vi "Clear Mutation History.vi"   [LabVIEW 2019]
uses:
  <vilib>/Utility/EditLVLibs/Edit LVLibs.lvlib
types:
  T1 = typedef "Edit LVLibs.lvlib/Mutation History.ctl" = T2[]
  T2 = typedef "Edit LVLibs.lvlib/Mutation Record.ctl" = cluster{"Library Version":T3, "Old Name Index":u8, "Class Default Data":variant, "Cluster Order Map":u32[], "Parent Name":string, "Parent Path":path, "LabVIEW Version":u32, "User Comments":string, "Mutation Flags":u8, "Parent Old Name Index":u8, "Parent Levels Added":u16, "Parent Levels Removed":u16}
  T3 = typedef "Edit LVLibs.lvlib/LibVersion.ctl" = cluster{"Major":u16, "Minor":u16, "Fix":u16, "Build":u16}
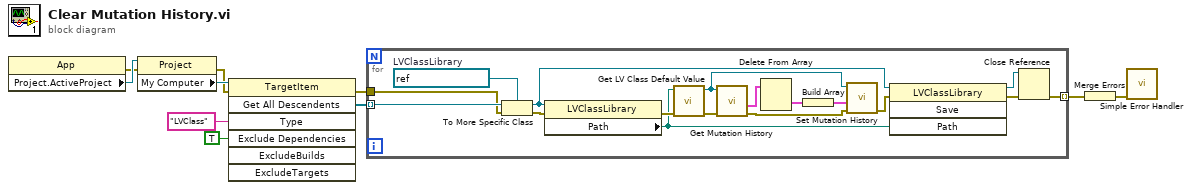
[diagram p0: block diagram]
diagram:
  n1 = property class="App"() -> (error out=w7:errorcluster, "Project.ActiveProject"=w10:refnum<vi>)  [unwired: 2 in, 1 out]
  n2 = property class="Project"(reference=w10, error in=w7) -> (error out=w6:errorcluster, "My Computer"=w9:refnum<vi>)  [unwired: 1 out]
  n3 = invoke class="TargetItem" method="Get All Descendents"(reference=w9, error in=w6, "Type"="LVClass", "Exclude Dependencies"=TRUE ("ExcludeDependencies")) -> (error out=w5:errorcluster, "All Descendents"=w4:refnum<vi>[])  [unwired: 3 in, 5 out]
  n4 = for {
    tunnel: w4 -> [w27] mode=indexing
    tunnel: w5 -> [w26]
    tunnel: [w18] -> w3 mode=indexing
    w25 = refnum<vi> refnum  # LVClassLibrary
    n5 = To More Specific Class(target class=w25, reference=w27, error in=w26) -> (specific class reference=w23:refnum<vi>, error out=w24:errorcluster)
    n6 = property class="LVClassLibrary"(reference=w23, error in=w24) -> (error out=w22:errorcluster, "Path"=w19:path)  [unwired: 1 out]
    n7 = call <vilib>:"Get LV Class Default Value.vi"("error in (no error)"=w22, "class path"=w19) -> ("error out"=w15:errorcluster, "object"=w16:refnum<class>)  [unwired: 8 in]
    n8 = call <vilib>:"Get Mutation History.vi"("error in"=w15, "Input object"=w16) -> ("error out"=w14:errorcluster, "Mutation History"=w13:T1)  [unwired: 6 in]
    n9 = Delete From Array(array=w13) -> (deleted portion=w12:T2)  [unwired: 2 in, 1 out]
    n10 = Build Array(w12) -> (w11:T2[])
    n11 = call <vilib>:"Set Mutation History.vi"("error in"=w14, "Mutation History"=w11, "Input object"=w16) -> ("error out"=w21:errorcluster)  [unwired: 8 in]
    n12 = invoke class="LVClassLibrary" method="Save"(reference=w23, error in=w21, "Path"=w19) -> (reference out=w17:refnum<vi>, error out=w20:errorcluster)  [unwired: 1 in, 2 out]
    n13 = Close Reference(reference=w17, error in (no error)=w20) -> (error out=w18:errorcluster)
  }
  n14 = Merge Errors(w3) -> (w2:errorcluster)
  n15 = call <vilib>:"Simple Error Handler.vi"("error in (no error)"=w2) -> ()  [unwired: 4 in, 5 out]
